vi "Get ni_measurements_v1_GetMetadataResponse.vi"(8 "error in (no error)":errorcluster, 11 "gRPCid":T8) -> (0 "error out":errorcluster, 2 "package_templatemessage":T1, 3 "gRPCid out":T8)   [LabVIEW 2020, in "LineRegulation.lvlib"]
uses:
  LineRegulation.lvlib
  <vilib>/gRPC/LabVIEW gRPC Library/Server API/typeDefs/grpcId.ctl
  ni_measurements_v1_GetMetadataResponse.ctl
  ni_measurements_v1_MeasurementDetails.ctl
  ni_measurements_v1_MeasurementParameters.ctl
  ni_measurements_v1_ConfigurationParameter.ctl
  google_protobuf_Any.ctl
  ni_measurements_v1_Output.ctl
  ni_measurements_v1_UserInterfaceDetails.ctl
  a51dd2a7-b5c1-4c09-9df4-8cd9d3bd0c19.vi
  <vilib>/gRPC/LabVIEW gRPC Library/Server API/Server/Get Server DLL Path.vi
  <vilib>/gRPC/LabVIEW gRPC Library/gprc-lvsupport-release.lvlib
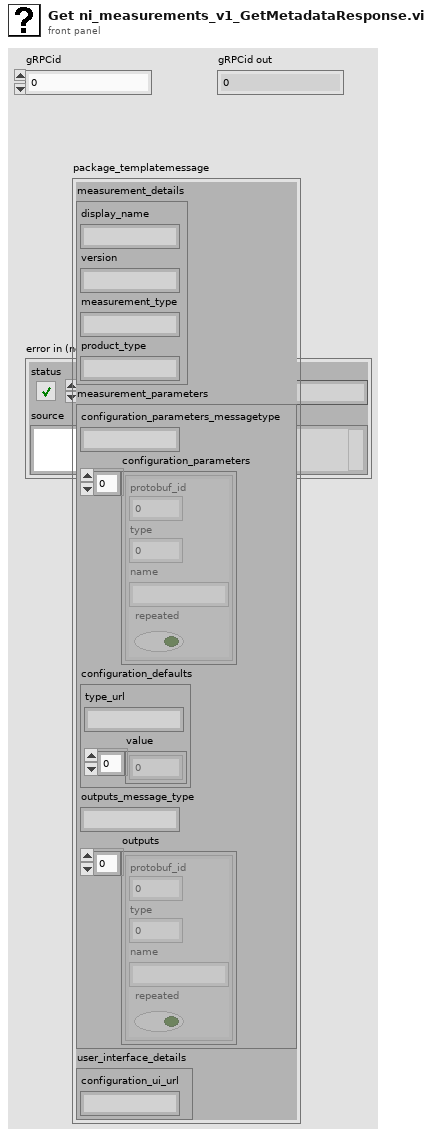
[diagram p1: front panel]
types:
  T1 = typedef "LineRegulation.lvlib/ni_measurements_v1_GetMetadataResponse.ctl" = cluster{"measurement_details":T2, "measurement_parameters":T3, "user_interface_details":T7}
  T2 = typedef "LineRegulation.lvlib/ni_measurements_v1_MeasurementDetails.ctl" = cluster{"display_name":string, "version":string, "measurement_type":string, "product_type":string}
  T3 = typedef "LineRegulation.lvlib/ni_measurements_v1_MeasurementParameters.ctl" = cluster{"configuration_parameters_messagetype":string, "configuration_parameters":T4[], "configuration_defaults":T5, "outputs_message_type":string, "outputs":T6[]}
  T4 = typedef "LineRegulation.lvlib/ni_measurements_v1_ConfigurationParameter.ctl" = cluster{"protobuf_id":u32, "type":i32, "name":string, "repeated":bool}
  T5 = typedef "LineRegulation.lvlib/google_protobuf_Any.ctl" = cluster{"type_url":string, "value":u8[]}
  T6 = typedef "LineRegulation.lvlib/ni_measurements_v1_Output.ctl" = cluster{"protobuf_id":u32, "type":i32, "name":string, "repeated":bool}
  T7 = typedef "LineRegulation.lvlib/ni_measurements_v1_UserInterfaceDetails.ctl" = cluster{"configuration_ui_url":string}
  T8 = typedef "gprc-lvsupport-release.lvlib/grpcId.ctl" = u64
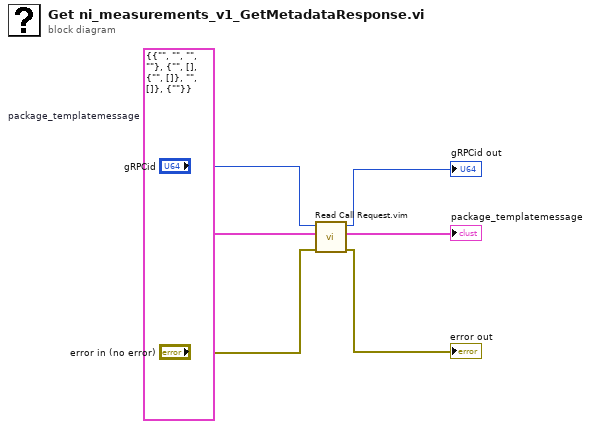
[diagram p0: block diagram]
diagram:
  w2 = T1 {"measurement_details"={"display_name"="", "version"="", "measurement_type"="", "product_type"=""}, "measurement_parameters"={"configuration_parameters_messagetype"="", "configuration_parameters"=[], "configuration_defaults"={"type_url"="", "value"=[]}, "outputs_message_type"="", "outputs"=[]}, "user_interface_details"={"configuration_ui_url"=""}}  # package_templatemessage
  n1 = call "Read Call Request.vim"("error in (no error)"="error in (no error)", "Data Type"=w2, "gRPCid in"="gRPCid") -> ("error out"=→"error out":errorcluster, "Request Data"=→"package_templatemessage":T1, "gRPCid out"=→"gRPCid out":T8)  [unwired: 6 in]
